vi "Init.vi"(8 "error in (no error)":errorcluster, 10 "Channel":i16=-10, 11 "AODAcq in":refnum<class "AODAcq.lvclass">) -> (0 "error out":errorcluster, 3 "AODAcq out":refnum<class "AODAcq.lvclass">)   [LabVIEW 2011, in "AODAcq.lvclass"]
uses:
  AODAcq.lvclass
  <vilib>/userdefined/High Color/nirio_resource_hc.ctl
  AcquistionObject/AcquistionObject.lvclass
  <vilib>/LabVIEW Targets/FPGA/RIO/nirio_PxiTriggers.ctl
  <vilib>/FPGAPlugInAG/PXIe-7965R/niLvFpga_Open_PXIe-7965R.vi
  <vilib>/FPGAPlugInAG/PXIe-7965R/niLvFpga_Reset_PXIe-7965R.vi
  <vilib>/FPGAPlugInAG/PXIe-7965R/niLvFpga_Run_PXIe-7965R.vi
  <vilib>/LabVIEW Targets/FPGA/RIO/nirioReserveTrigger.vi
  <vilib>/LabVIEW Targets/FPGA/79XXR/Private/79XXR_Method_IOModuleStatusImpl.vi
  <vilib>/Utility/error.llb/Error Cluster From Error Code.vi
  <vilib>/rvi/errors/niLvFpgaAdjustHostInterfaceError.vi
  <vilib>/rvi/interface/nirviOpenFPGA/nirviOpenFPGA.xnode
  FPGA_Control/AODRef.ctl
  FPGA Bitfiles/Acquisition_FPGATarget_AODControl(FPGA)_C1C38267.lvbitx
  FPGA_Control/AOD Control (FPGA).vi
  <vilib>/rvi/interface/nirviMethod/nirviMethod.xnode
  <vilib>/FPGA/interface/niFpgaViExecutionMode.ctl
  <vilib>/rvi/interface/nirviReadWriteControl/nirviReadWriteControl.xnode
  NiFpgaLv.dll
  <vilib>/FPGAPlugInAG/PXIe-7965R/niLvFpga_ConfigureFifo_PXIe-7965R.vi
  <vilib>/rvi/errors/niLvFpgaMergeErrorWithErrorCode.vi
  <vilib>/FPGAPlugInAG/PXIe-7965R/niLvFpga_StartFifo_PXIe-7965R.vi
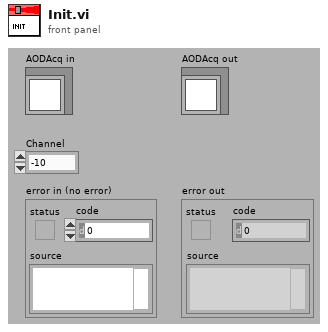
[diagram p1: front panel]
types:
  T1 = typedef "nirio_resource_hc.ctl" = tag
  T2 = typedef "AODRef.ctl" = refnum<k20>
  T3 = typedef "niFpgaViExecutionMode.ctl" = enum16{"FPGA Target", "Development Computer with Simulated I/O", "Development Computer with Real I/O", "Third-Party Simulator"}
  T4 = typedef "nirio_PxiTriggers.ctl" = u16
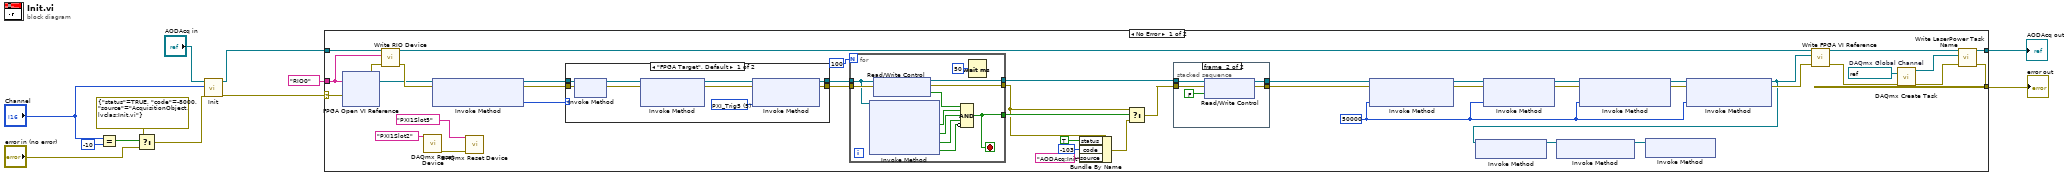
[diagram p0: block diagram]
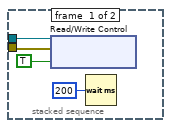
[diagram p2: hidden frame]
diagram:
  n1 = Equal?(x="Channel", y=i16 -10 ("x")) -> (x = y?=w8:bool)
  n2 = Select(t=errorcluster {"status"=TRUE, "code"=-8000, "source"="AcquisitionObject.lvclas:Init.vi"}, s=w8, f="error in (no error)") -> (s? t:f=w3:errorcluster)
  n3 = call-parent "Init.vi"("error in (no error)"=w3, "Channel"="Channel", "AcquistionObject in"="AODAcq in") -> ("error out"=w2:errorcluster, "AcquistionObject out"=w1:refnum<class "AODAcq.lvclass">)  [unwired: 7 in]
  n4 = case shown="No Error" w2 {
    selector: w2 -> [w54 w89]
    tunnel: [w45 w89] -> w12
    tunnel: [w46 w88] -> w11
    tunnel: w1 -> [w44 w88]
    tunnel: T1 "RIO0" ("RIO Device") -> [w42 _]
    frame No Error {
      w51 = refnum<k21> "AOD Gain"  # DAQmx Global Channel
      w19 = u32 50000 ("Depth")
      n5 = xnode "FPGA Open VI Reference"("error in"=w54, "resource name"=w42) -> ("FPGA VI Reference Out"=w39:T2, "error out"=w41:errorcluster)
      n6 = call-dynamic "Write RIO Device.vi"("error in (no error)"=w41, "RIO Device"=w42, "AODAcq in"=w44) -> ("error out"=w40:errorcluster, "AODAcq out"=w43:refnum<class "AODAcq.lvclass">)  [unwired: 7 in]
      n7 = call <vilib>:"DAQmx Reset Device.vi"("device in"=tag "PXI1Slot2") -> ("error out"=w26:errorcluster)  [unwired: 14 in]
      n8 = xnode "Invoke Method"("FPGA VI Reference In"=w39, "error in"=w40) -> ("FPGA VI Reference Out"=w56:T2, "error out"=w53:errorcluster, "FPGA VI Execution Mode"=w55:T3)
      n9 = call <vilib>:"DAQmx Reset Device.vi"("device in"=tag "PXI1Slot5", "error in"=w26) -> ()  [unwired: 13 in, 1 out]
      n10 = case shown="\"FPGA Target\", Default" w55 {
        tunnel: [w81 w87] -> w38
        tunnel: w56 -> [w85 w87]
        tunnel: w53 -> [w80 w86]
        tunnel: [w77 w86] -> w37
        frame "FPGA Target", Default {
          w83 = T4 5 items=["PXI_Trig0", "PXI_Trig1", "PXI_Trig2", "PXI_Trig3", "PXI_Trig4", "PXI_Trig5", "PXI_Trig6", "PXI_Trig7"] ("Trigger")
          n11 = xnode "Invoke Method"("FPGA VI Reference In"=w85, "error in"=w80) -> ("FPGA VI Reference Out"=w84:T2, "error out"=w79:errorcluster)
          n12 = xnode "Invoke Method"("FPGA VI Reference In"=w84, "error in"=w79) -> ("FPGA VI Reference Out"=w82:T2, "error out"=w78:errorcluster)  [unwired: 1 in]
          n13 = xnode "Invoke Method"("FPGA VI Reference In"=w82, "error in"=w78, "Trigger"=w83) -> ("FPGA VI Reference Out"=w81:T2, "error out"=w77:errorcluster)
        }
        frame "Development Computer with Simulated I/O" {
        }
      }
      n14 = for {
        N: 100 -> [_]
        tunnel: w38 -> [w66]
        tunnel: w37 -> [w67]
        tunnel: [w58] -> w36
        tunnel: [w60] -> w34
        tunnel: [w57] -> w29
        stop <- w58 stop-if-true
        n15 = xnode "Invoke Method"("FPGA VI Reference In"=w66) -> ("IO Module Present?"=w64:bool, "Power Enabled?"=w63:bool, "IO Enabled?"=w62:bool, "IO Module Mismatch?"=w61:bool)  [unwired: 1 in, 2 out]
        n16 = xnode "Read/Write Control"("FPGA VI Reference In"=w66, "error in"=w67) -> ("FPGA VI Reference Out"=w57:T2, "error out"=w60:errorcluster, "Status.Initialized"=w65:bool)
        n17 = Compound Arithmetic op=AND(w65, w64, w63, w62, invert w61) -> (w58:bool)
        n18 = Wait (ms)(milliseconds to wait=u32 50) -> ()  [unwired: 1 out]
      }
      n19 = Bundle By Name(cluster=w34, "status"=TRUE, "code"=-103, "source"="AODAcq:Init") -> (w33:errorcluster)
      n20 = Select(t=w34, s=w36, f=w33) -> (s? t:f=w28:errorcluster)
      n21 = stacked-sequence {
        tunnel: w29 -> [w71 w76]
        tunnel: w28 -> [w70 w75]
        tunnel: [_ w73] -> w14
        tunnel: [_ w72] -> w13
        frame #0 {
          n22 = xnode "Read/Write Control"("FPGA VI Reference In"=w71, "error in"=w70, "Control.Reset"=TRUE) -> ()  [unwired: 2 out]
          n23 = Wait (ms)(milliseconds to wait=u32 200) -> ()  [unwired: 1 out]
        }
        frame #1 {
          n24 = xnode "Read/Write Control"("FPGA VI Reference In"=w76, "error in"=w75, "Control.Reset"=FALSE) -> ("FPGA VI Reference Out"=w73:T2, "error out"=w72:errorcluster)
        }
      }
      n25 = xnode "Invoke Method"("FPGA VI Reference In"=w14, "error in"=w13, "Depth"=w19) -> ("FPGA VI Reference Out"=w18:T2, "error out"=w52:errorcluster)
      n26 = xnode "Invoke Method"("FPGA VI Reference In"=w18, "error in"=w52, "Depth"=w19) -> ("FPGA VI Reference Out"=w24:T2, "error out"=w23:errorcluster)
      n27 = xnode "Invoke Method"("FPGA VI Reference In"=w24, "error in"=w23, "Depth"=w19) -> ("FPGA VI Reference Out"=w22:T2, "error out"=w21:errorcluster)
      n28 = xnode "Invoke Method"("FPGA VI Reference In"=w22, "error in"=w21, "Depth"=w19) -> ("FPGA VI Reference Out"=w17:T2, "error out"=w20:errorcluster)
      n29 = xnode "Invoke Method"("FPGA VI Reference In"=w17) -> ("FPGA VI Reference Out"=w16:T2)  [unwired: 1 in, 1 out]
      n30 = xnode "Invoke Method"("FPGA VI Reference In"=w16) -> ("FPGA VI Reference Out"=w15:T2)  [unwired: 1 in, 1 out]
      n31 = xnode "Invoke Method"("FPGA VI Reference In"=w15) -> ()  [unwired: 1 in, 2 out]
      n32 = call-dynamic "Write FPGA VI Reference.vi"("error in (no error)"=w20, "AOD FPGA"=w17, "AODAcq in"=w43) -> ("error out"=w50:errorcluster, "AODAcq out"=w47:refnum<class "AODAcq.lvclass">)  [unwired: 7 in]
      n33 = call <vilib>:"DAQmx Create Task.vi"("global virtual channels"=w51, "error in"=w50) -> ("task out"=w48:refnum<k21>, "error out"=w49:errorcluster)  [unwired: 3 in, 9 out]
      n34 = call-dynamic "Write LaserPower Task Name.vi"("error in (no error)"=w49, "LaserPower Task Name"=w48, "AODAcq in"=w47) -> ("error out"=w45:errorcluster, "AODAcq out"=w46:refnum<class "AODAcq.lvclass">)  [unwired: 7 in]
    }
    frame Error {
    }
  }
  "error out" <- w12
  "AODAcq out" <- w11
